vi "Read and Return AO Task.vi"(0 "OSC Configuration In":T1(array[cluster])=[[{"Signal Type"=enum."Sine Wave", "DC"=0.0, "Amplitude"=0.01, "frequency"=2.0, "Phase"=0.0}, {"Signal Type"=enum."Sine Wave", "DC"=0.0, "Amplitude"=0.01, "frequency"=2.0, "Phase"=0.0}], [{"Signal Type"=enum."Sine Wave", "DC"=0.0, "Amplitude"=0.01, "frequency"=2.0, "Phase"=0.0}, {"Signal Type"=enum."Sine Wave", "DC"=0.0, "Amplitude"=0.01, "frequency"=2.0, "Phase"=0.0}]] {"frequency" step=0.001 format="%.3p"; "Amplitude" format="%0.2p"; "DC" min=-0.99 max=0.99 format="%.2p"}, 1 "AO Task In":refnum<k21>[](array[refnum])=[""], 2 "Sampling Information In":cluster{"Fs":dbl, "#s":dbl}[](array[cluster])=[{"Fs"=10000.0, "#s"=5000.0}, {"Fs"=10000.0, "#s"=5000.0}], 3 "Multiplication Factor In":dbl=1.0) -> ()   [LabVIEW 2013, in "Lock-In Variable Channels_2.lvclass"]
uses:
  Lock-In Variable Channels_2.lvclass
  <vilib>/DAQmx/write.llb/DAQmx Write (Analog 1D Wfm NChan NSamp).vi
  <vilib>/DAQmx/miscellaneous.llb/DAQmx Fill In Error Info.vi
panel:
  in  "OSC Configuration Control":T1(array[cluster])=[[{"Signal Type"=enum."Sine Wave", "DC"=0.0, "Amplitude"=0.001, "frequency"=2.0, "Phase"=0.0}, {"Signal Type"=enum."Sine Wave", "DC"=0.0, "Amplitude"=0.0, "frequency"=2.0, "Phase"=0.0}, {"Signal Type"=enum."Sine Wave", "DC"=0.0, "Amplitude"=0.0, "frequency"=20.0, "Phase"=0.0}], [{"Signal Type"=enum."Sine Wave", "DC"=0.0, "Amplitude"=0.0, "frequency"=2.0, "Phase"=0.0}, {"Signal Type"=enum."Sine Wave", "DC"=0.0, "Amplitude"=0.0, "frequency"=2.0, "Phase"=0.0}, {"Signal Type"=enum."Sine Wave", "DC"=0.0, "Amplitude"=0.0, "frequency"=20.0, "Phase"=0.0}]] {"frequency" step=0.001 format="%.3p"; "Amplitude" format="%0.2p"; "DC" min=-0.99 max=0.99 format="%.2p"}
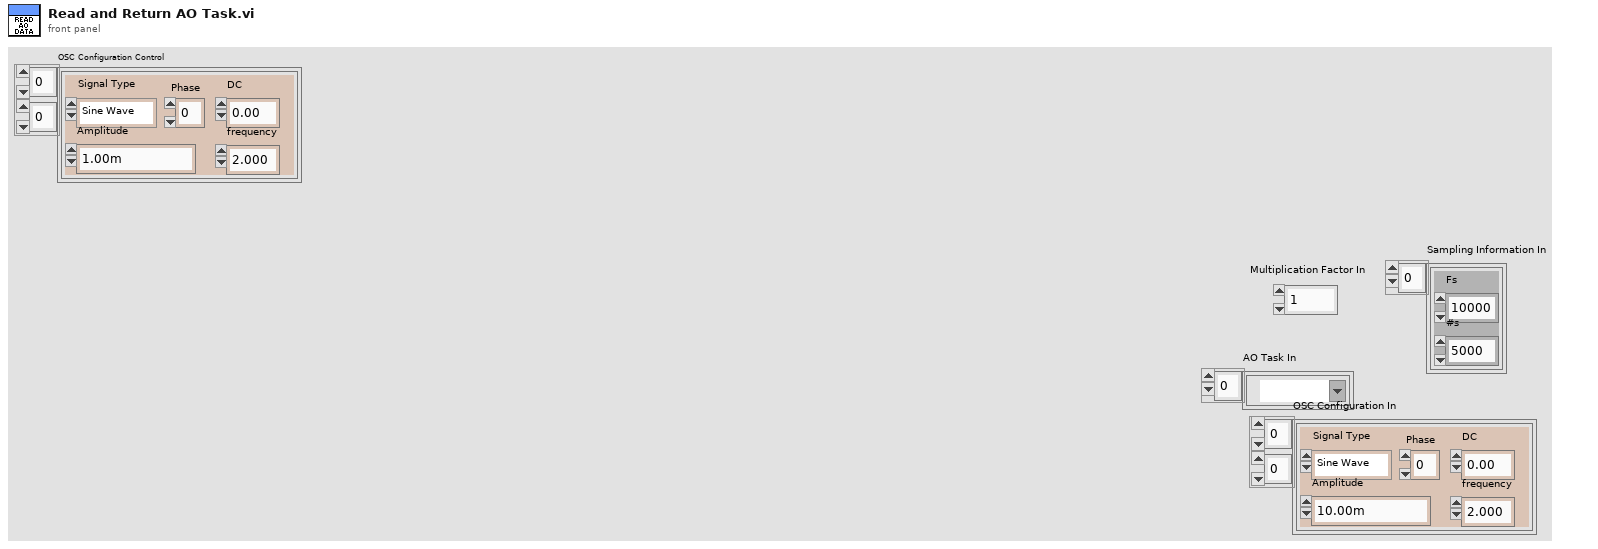
[diagram p1: front panel]
types:
  T1 = cluster{"Signal Type":enum16{"Sine Wave", "Triangle Wave", "Square Wave", "Sawtooth Wave"}, "DC":dbl, "Amplitude":dbl, "frequency":dbl, "Phase":dbl}[][]
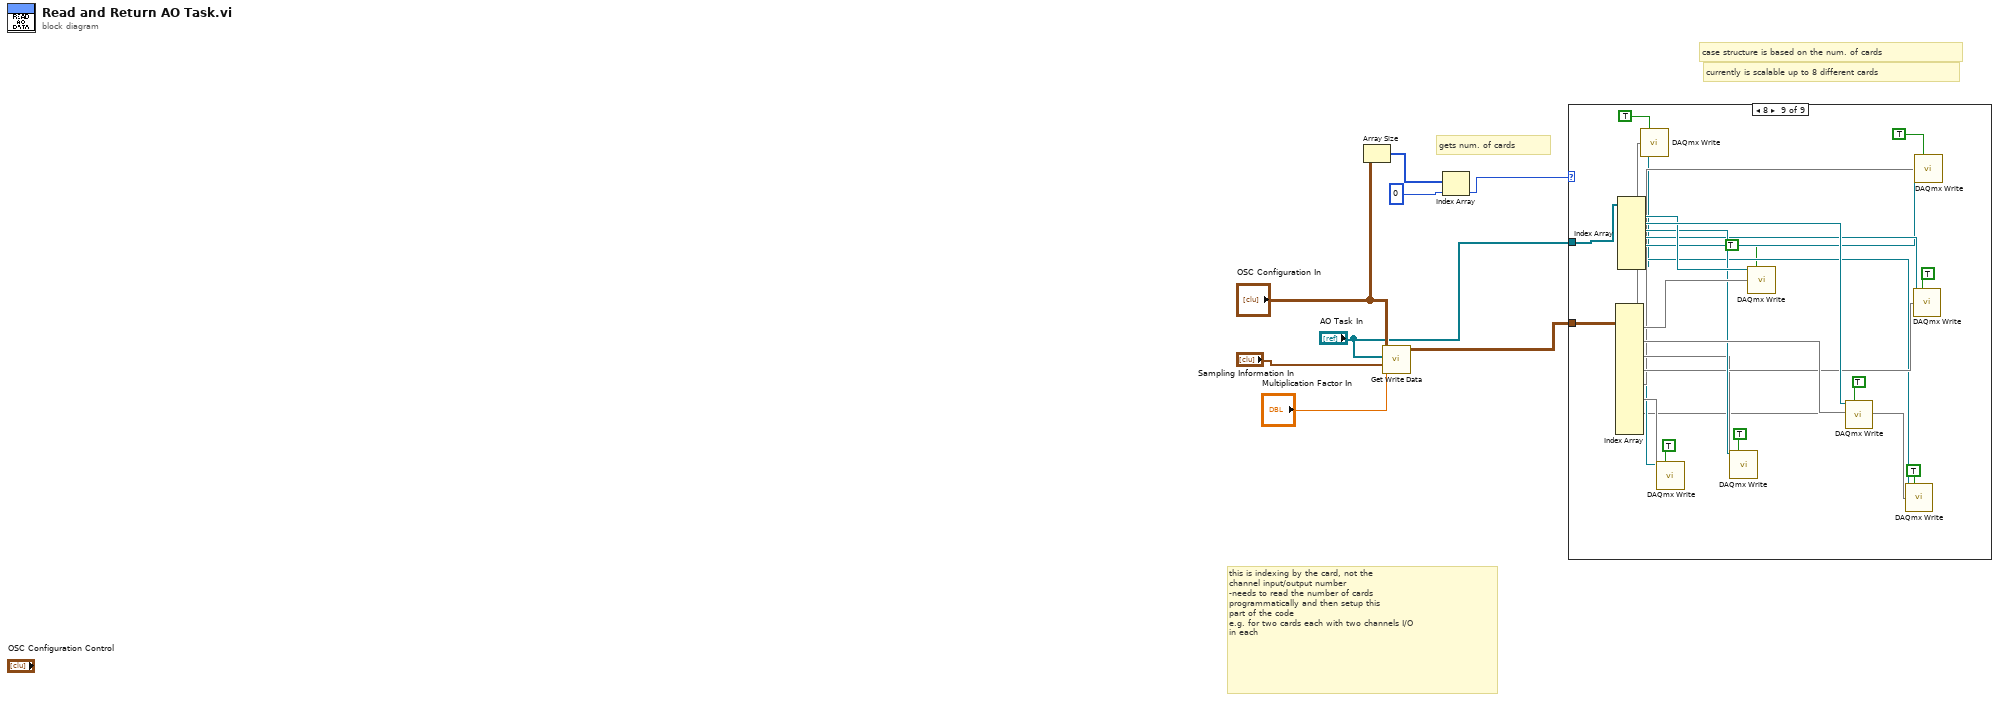
[diagram p0: block diagram]
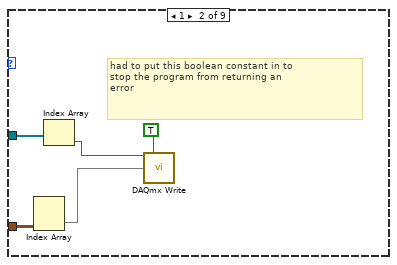
[diagram p3: hidden frame]
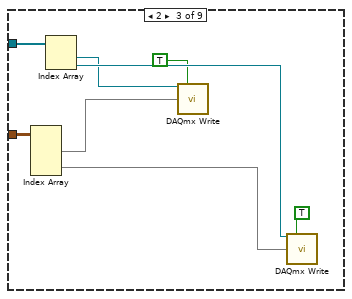
[diagram p4: hidden frame]
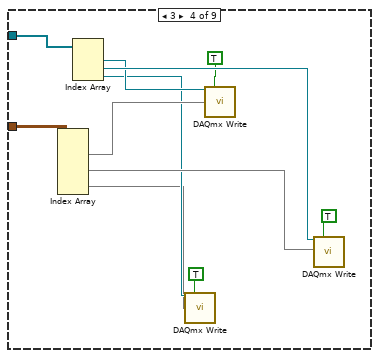
[diagram p5: hidden frame]
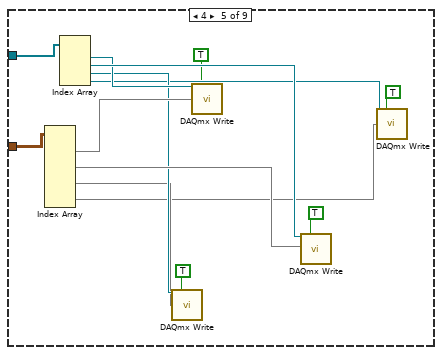
[diagram p6: hidden frame]
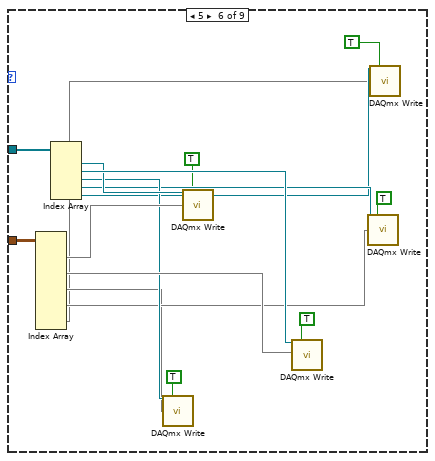
[diagram p7: hidden frame]
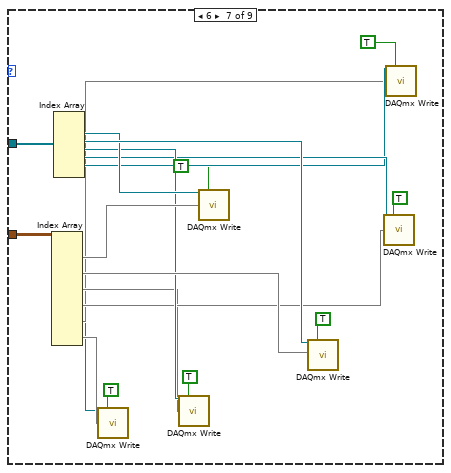
[diagram p8: hidden frame]
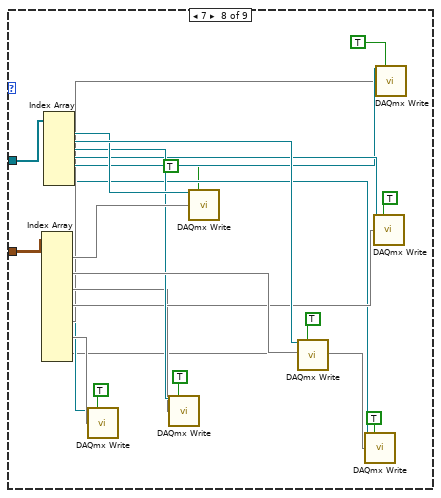
[diagram p9: hidden frame]
diagram:
  # "currently is scalable up to 8 different cards"
  # "case structure is based on the num. of cards"
  # "gets num. of cards"
  # "this is indexing by the card, not the\nchannel input/output number\n-needs to read the number of cards\nprogrammatically and then setup this\npart of the code\ne.g. for two cards each with two channels I/O\nin each"
  n1 = Array Size(array="OSC Configuration In") -> (size(s)=w5:i32[])
  n2 = call "Get Write Data.vi"("Multiplication Factor"="Multiplication Factor In", "Sampling information 2"="Sampling Information In", "AO Task"="AO Task In", "OSC Configuration"="OSC Configuration In") -> ("Data"=w2:waveform(dbl)[][])  [unwired: 7 in]
  n3 = Index Array(array=w5, index=0) -> (element=w3:i32)
  n4 = case shown="8" w3 {
    tunnel: w2 -> [_ w11 w16 w27 w37 w52 w68 w88 w111]
    tunnel: "AO Task In" -> [_ w13 w15 w28 w38 w53 w69 w89 w112]
    frame 0, Default {
    }
    frame 1 {
      # "had to put this boolean constant in to\nstop the program from returning an\nerror"
      n5 = Index Array(array=w11) -> (element=w10:waveform(dbl)[])  [unwired: 2 in]
      n6 = Index Array(array=w13) -> (element=w12:refnum<k21>)  [unwired: 1 in]
      n7 = call-poly <vilib>:"DAQmx Write.vi"("task/channels in"=w12, "auto start"=TRUE, "data"=w10) -> ()  [unwired: 10 in, 3 out]
    }
    frame 2 {
      n8 = Index Array(array=w16) -> (element #1=w17:waveform(dbl)[], element #2=w18:waveform(dbl)[])  [unwired: 4 in]
      n9 = Index Array(array=w15) -> (element #1=w19:refnum<k21>, element #2=w20:refnum<k21>)  [unwired: 2 in]
      n10 = call-poly <vilib>:"DAQmx Write.vi"("task/channels in"=w19, "auto start"=TRUE, "data"=w17) -> ()  [unwired: 10 in, 3 out]
      n11 = call-poly <vilib>:"DAQmx Write.vi"("task/channels in"=w20, "auto start"=TRUE, "data"=w18) -> ()  [unwired: 10 in, 3 out]
    }
    frame 3 {
      n12 = Index Array(array=w27) -> (element #1=w29:waveform(dbl)[], element #2=w26:waveform(dbl)[], element #3=w24:waveform(dbl)[])  [unwired: 6 in]
      n13 = Index Array(array=w28) -> (element #1=w30:refnum<k21>, element #2=w31:refnum<k21>, element #3=w25:refnum<k21>)  [unwired: 3 in]
      n14 = call-poly <vilib>:"DAQmx Write.vi"("task/channels in"=w25, "auto start"=TRUE, "data"=w24) -> ()  [unwired: 10 in, 3 out]
      n15 = call-poly <vilib>:"DAQmx Write.vi"("task/channels in"=w30, "auto start"=TRUE, "data"=w29) -> ()  [unwired: 10 in, 3 out]
      n16 = call-poly <vilib>:"DAQmx Write.vi"("task/channels in"=w31, "auto start"=TRUE, "data"=w26) -> ()  [unwired: 10 in, 3 out]
    }
    frame 4 {
      n17 = Index Array(array=w37) -> (element #1=w43:waveform(dbl)[], element #2=w42:waveform(dbl)[], element #3=w40:waveform(dbl)[], element #4=w35:waveform(dbl)[])  [unwired: 8 in]
      n18 = Index Array(array=w38) -> (element #1=w44:refnum<k21>, element #2=w45:refnum<k21>, element #3=w41:refnum<k21>, element #4=w36:refnum<k21>)  [unwired: 4 in]
      n19 = call-poly <vilib>:"DAQmx Write.vi"("task/channels in"=w41, "auto start"=TRUE, "data"=w40) -> ()  [unwired: 10 in, 3 out]
      n20 = call-poly <vilib>:"DAQmx Write.vi"("task/channels in"=w44, "auto start"=TRUE, "data"=w43) -> ()  [unwired: 10 in, 3 out]
      n21 = call-poly <vilib>:"DAQmx Write.vi"("task/channels in"=w45, "auto start"=TRUE, "data"=w42) -> ()  [unwired: 10 in, 3 out]
      n22 = call-poly <vilib>:"DAQmx Write.vi"("task/channels in"=w36, "auto start"=TRUE, "data"=w35) -> ()  [unwired: 10 in, 3 out]
    }
    frame 5 {
      n23 = Index Array(array=w52) -> (element #1=w60:waveform(dbl)[], element #2=w59:waveform(dbl)[], element #3=w51:waveform(dbl)[], element #4=w55:waveform(dbl)[], element #5=w49:waveform(dbl)[])  [unwired: 10 in]
      n24 = Index Array(array=w53) -> (element #1=w61:refnum<k21>, element #2=w62:refnum<k21>, element #3=w58:refnum<k21>, element #4=w56:refnum<k21>, element #5=w50:refnum<k21>)  [unwired: 5 in]
      n25 = call-poly <vilib>:"DAQmx Write.vi"("task/channels in"=w58, "auto start"=TRUE, "data"=w51) -> ()  [unwired: 10 in, 3 out]
      n26 = call-poly <vilib>:"DAQmx Write.vi"("task/channels in"=w61, "auto start"=TRUE, "data"=w60) -> ()  [unwired: 10 in, 3 out]
      n27 = call-poly <vilib>:"DAQmx Write.vi"("task/channels in"=w62, "auto start"=TRUE, "data"=w59) -> ()  [unwired: 10 in, 3 out]
      n28 = call-poly <vilib>:"DAQmx Write.vi"("task/channels in"=w56, "auto start"=TRUE, "data"=w55) -> ()  [unwired: 10 in, 3 out]
      n29 = call-poly <vilib>:"DAQmx Write.vi"("task/channels in"=w50, "auto start"=TRUE, "data"=w49) -> ()  [unwired: 10 in, 3 out]
    }
    frame 6 {
      n30 = Index Array(array=w68) -> (element #1=w80:waveform(dbl)[], element #2=w79:waveform(dbl)[], element #3=w73:waveform(dbl)[], element #4=w75:waveform(dbl)[], element #5=w71:waveform(dbl)[], element #6=w66:waveform(dbl)[])  [unwired: 12 in]
      n31 = Index Array(array=w69) -> (element #1=w81:refnum<k21>, element #2=w82:refnum<k21>, element #3=w78:refnum<k21>, element #4=w76:refnum<k21>, element #5=w72:refnum<k21>, element #6=w65:refnum<k21>)  [unwired: 6 in]
      n32 = call-poly <vilib>:"DAQmx Write.vi"("task/channels in"=w65, "auto start"=TRUE, "data"=w66) -> ()  [unwired: 10 in, 3 out]
      n33 = call-poly <vilib>:"DAQmx Write.vi"("task/channels in"=w78, "auto start"=TRUE, "data"=w73) -> ()  [unwired: 10 in, 3 out]
      n34 = call-poly <vilib>:"DAQmx Write.vi"("task/channels in"=w81, "auto start"=TRUE, "data"=w80) -> ()  [unwired: 10 in, 3 out]
      n35 = call-poly <vilib>:"DAQmx Write.vi"("task/channels in"=w82, "auto start"=TRUE, "data"=w79) -> ()  [unwired: 10 in, 3 out]
      n36 = call-poly <vilib>:"DAQmx Write.vi"("task/channels in"=w76, "auto start"=TRUE, "data"=w75) -> ()  [unwired: 10 in, 3 out]
      n37 = call-poly <vilib>:"DAQmx Write.vi"("task/channels in"=w72, "auto start"=TRUE, "data"=w71) -> ()  [unwired: 10 in, 3 out]
    }
    frame 7 {
      n38 = Index Array(array=w88) -> (element #1=w103:waveform(dbl)[], element #2=w102:waveform(dbl)[], element #3=w96:waveform(dbl)[], element #4=w98:waveform(dbl)[], element #5=w94:waveform(dbl)[], element #6=w91:waveform(dbl)[], element #7=w86:waveform(dbl)[])  [unwired: 14 in]
      n39 = Index Array(array=w89) -> (element #1=w104:refnum<k21>, element #2=w105:refnum<k21>, element #3=w101:refnum<k21>, element #4=w99:refnum<k21>, element #5=w95:refnum<k21>, element #6=w90:refnum<k21>, element #7=w85:refnum<k21>)  [unwired: 7 in]
      n40 = call-poly <vilib>:"DAQmx Write.vi"("task/channels in"=w90, "auto start"=TRUE, "data"=w91) -> ()  [unwired: 10 in, 3 out]
      n41 = call-poly <vilib>:"DAQmx Write.vi"("task/channels in"=w101, "auto start"=TRUE, "data"=w96) -> ()  [unwired: 10 in, 3 out]
      n42 = call-poly <vilib>:"DAQmx Write.vi"("task/channels in"=w104, "auto start"=TRUE, "data"=w103) -> ()  [unwired: 10 in, 3 out]
      n43 = call-poly <vilib>:"DAQmx Write.vi"("task/channels in"=w105, "auto start"=TRUE, "data"=w102) -> ()  [unwired: 10 in, 3 out]
      n44 = call-poly <vilib>:"DAQmx Write.vi"("task/channels in"=w85, "auto start"=TRUE, "data"=w86) -> ()  [unwired: 10 in, 3 out]
      n45 = call-poly <vilib>:"DAQmx Write.vi"("task/channels in"=w99, "auto start"=TRUE, "data"=w98) -> ()  [unwired: 10 in, 3 out]
      n46 = call-poly <vilib>:"DAQmx Write.vi"("task/channels in"=w95, "auto start"=TRUE, "data"=w94) -> ()  [unwired: 10 in, 3 out]
    }
    frame 8 {
      n47 = Index Array(array=w111) -> (element #1=w129:waveform(dbl)[], element #2=w128:waveform(dbl)[], element #3=w122:waveform(dbl)[], element #4=w124:waveform(dbl)[], element #5=w120:waveform(dbl)[], element #6=w117:waveform(dbl)[], element #7=w114:waveform(dbl)[], element #8=w108:waveform(dbl)[])  [unwired: 16 in]
      n48 = Index Array(array=w112) -> (element #1=w130:refnum<k21>, element #2=w131:refnum<k21>, element #3=w127:refnum<k21>, element #4=w125:refnum<k21>, element #5=w121:refnum<k21>, element #6=w116:refnum<k21>, element #7=w113:refnum<k21>, element #8=w109:refnum<k21>)  [unwired: 8 in]
      n49 = call-poly <vilib>:"DAQmx Write.vi"("task/channels in"=w109, "auto start"=TRUE, "data"=w108) -> ()  [unwired: 10 in, 3 out]
      n50 = call-poly <vilib>:"DAQmx Write.vi"("task/channels in"=w116, "auto start"=TRUE, "data"=w117) -> ()  [unwired: 10 in, 3 out]
      n51 = call-poly <vilib>:"DAQmx Write.vi"("task/channels in"=w127, "auto start"=TRUE, "data"=w122) -> ()  [unwired: 10 in, 3 out]
      n52 = call-poly <vilib>:"DAQmx Write.vi"("task/channels in"=w130, "auto start"=TRUE, "data"=w129) -> ()  [unwired: 10 in, 3 out]
      n53 = call-poly <vilib>:"DAQmx Write.vi"("task/channels in"=w131, "auto start"=TRUE, "data"=w128) -> ()  [unwired: 10 in, 3 out]
      n54 = call-poly <vilib>:"DAQmx Write.vi"("task/channels in"=w113, "auto start"=TRUE, "data"=w114) -> ()  [unwired: 10 in, 3 out]
      n55 = call-poly <vilib>:"DAQmx Write.vi"("task/channels in"=w125, "auto start"=TRUE, "data"=w124) -> ()  [unwired: 10 in, 3 out]
      n56 = call-poly <vilib>:"DAQmx Write.vi"("task/channels in"=w121, "auto start"=TRUE, "data"=w120) -> ()  [unwired: 10 in, 3 out]
    }
  }
